vi "Set Visible State.vi"(6 "Event Structure Frame (-1: Use State Name)":i32=-1, 7 "Event Structure (F: Case Structure)":bool, 8 "error in (no error)":errorcluster, 9 "State Name":string, 10 "Category (Optional)":string, 11 "JKI SM in":refnum<class "JKI SM.lvclass">) -> (0 "error out":errorcluster, 3 "JKI SM out":refnum<class "JKI SM.lvclass">)   [LabVIEW 2020, in "JKI State Machine API.lvlib" / "JKI SM.lvclass"]
uses:
  JKI SM.lvclass
  JKI SM.lvclass/JKI SM.ctl
  <userlib>/_OpenG.lib/string/string.llb/Trim Whitespace (String Array)__ogtk.vi
  <userlib>/_OpenG.lib/string/string.llb/Trim Whitespace (String)__ogtk.vi
  <userlib>/_OpenG.lib/string/string.llb/openg_string.lvlib
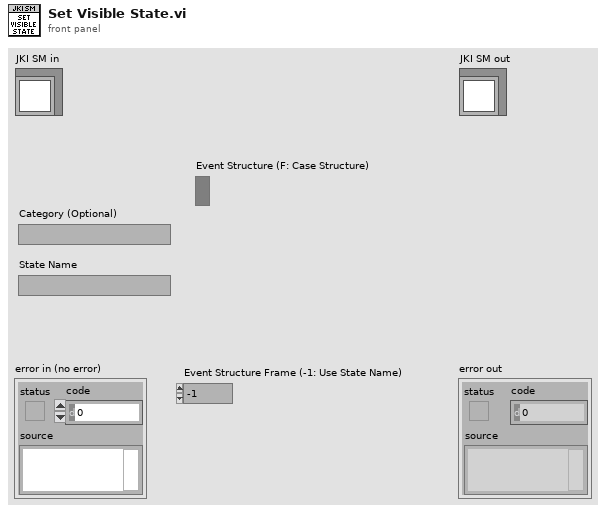
[diagram p1: front panel]
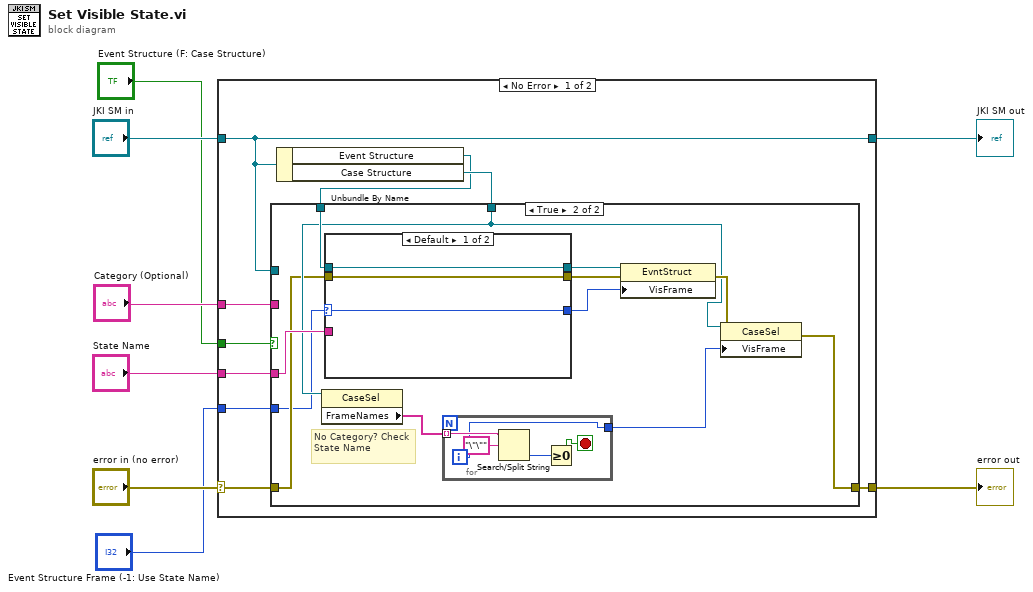
[diagram p0: block diagram]
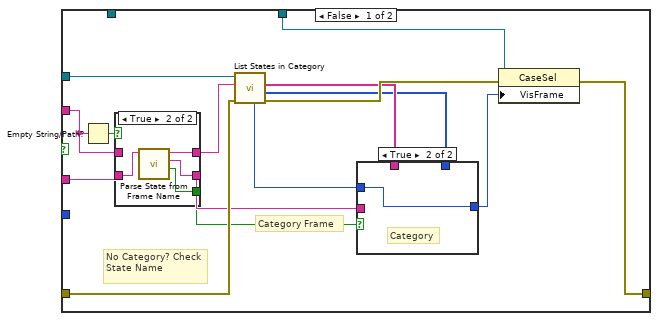
[diagram p2: hidden frame]
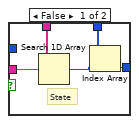
[diagram p3: hidden frame]
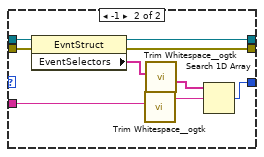
[diagram p5: hidden frame]
diagram:
  n1 = case shown="No Error" "error in (no error)" {
    selector: "error in (no error)" -> [w12 w75]
    tunnel: [w17 w75] -> w7
    tunnel: [w13 w74] -> w5
    tunnel: "JKI SM in" -> [w13 w74]
    tunnel: "State Name" -> [w14 _]
    tunnel: "Category (Optional)" -> [w15 _]
    tunnel: "Event Structure (F: Case Structure)" -> [w11 _]
    tunnel: "Event Structure Frame (-1: Use State Name)" -> [w9 _]
    frame No Error {
      n2 = Unbundle By Name(w13) -> ("Event Structure"=w10:refnum<vi>, "Case Structure"=w16:refnum<vi>)
      n3 = case shown="True" w11 {
        tunnel: [w32 w51] -> w17
        tunnel: w16 -> [w31 w50]
        tunnel: w15 -> [w28 _]
        tunnel: w14 -> [w27 w56]
        tunnel: w13 -> [w26 _]
        tunnel: w12 -> [w25 w47]
        tunnel: w10 -> [_ w54]
        tunnel: w9 -> [_ w45]
        frame False {
          # "Category Frame"
          # "No Category? Check State Name"
          n4 = Empty String/Path?(string/path=w28) -> (empty?=w29:bool)
          n5 = case shown="True" w29 {
            tunnel: w27 -> [w39 w44]
            tunnel: [w40 w43] -> w24
            tunnel: w28 -> [w40 _]
            tunnel: [w39 w42] -> w22
            tunnel: [_ w41] -> w19
            frame False {
            }
            frame True {
              n6 = call "Parse State from Frame Name.vi"("Frame or State Name"=w44) -> ("is a Category Frame?"=w41:bool, "State Name"=w42:string, "Category Name"=w43:string)  [unwired: 5 in, 3 out]
            }
          }
          n7 = call "List States in Category.vi"("error in (no error)"=w25, "Category"=w24, "JKI SM in"=w26) -> ("error out"=w30:errorcluster, "State Frame Indices"=w21:i32[], "States"=w23:string[], "Category Frame Index"=w18:i32)  [unwired: 4 in, 1 out]
          n8 = case shown="True" w19 {
            tunnel: w23 -> [w37 _]
            tunnel: w22 -> [w36 _]
            tunnel: w21 -> [w35 _]
            tunnel: [w33 w38] -> w20
            tunnel: w18 -> [_ w38]
            frame False {
              # "State"
              n9 = Search 1D Array(1D array=w37, element=w36) -> (index of element=w34:i32)  [unwired: 1 in]
              n10 = Index Array(array=w35, index=w34) -> (element=w33:i32)
            }
            frame True {
              # "Category"
            }
          }
          n11 = property class="CaseSel"(reference=w31, error in=w30, "VisFrame"=w20) -> (error out=w32:errorcluster)  [unwired: 1 out]
        }
        frame True {
          # "No Category? Check State Name"
          n12 = property class="CaseSel"(reference=w50) -> ("FrameNames"=w49:string[])  [unwired: 1 in, 2 out]
          n13 = case shown="Default" w45 {
            selector: w45 -> [w58 _]
            tunnel: w56 -> [_ w68]
            tunnel: [w58 w67] -> w55
            tunnel: w54 -> [w59 w66]
            tunnel: [w59 w64] -> w53
            tunnel: w47 -> [w57 w61]
            tunnel: [w57 w60] -> w46
            frame Default {
            }
            frame -1 {
              n14 = property class="EvntStruct"(reference=w66, error in=w61) -> (reference out=w64:refnum<vi>, error out=w60:errorcluster, "EventSelectors"=w65:string[])
              n15 = call-poly <userlib>:"Trim Whitespace__ogtk.vi"("String in"=w68) -> ("String out"=w62:string)  [unwired: 6 in]
              n16 = call-poly <userlib>:"Trim Whitespace__ogtk.vi"("String in"=w65) -> ("String out"=w63:string[])  [unwired: 6 in]
              n17 = Search 1D Array(1D array=w63, element=w62) -> (index of element=w67:i32)  [unwired: 1 in]
            }
          }
          n18 = for {
            tunnel: w49 -> [w73] mode=indexing
            tunnel: [w70] -> w48
            i -> [w70]
            stop <- w69 stop-if-true
            n19 = Search/Split String(string=w73, search string/char (-)="\"\"") -> (offset of match=w71:i32)  [unwired: 1 in, 2 out]
            n20 = Greater Or Equal To 0?(x=w71) -> (x >= 0?=w69:bool)
          }
          n21 = property class="EvntStruct"(reference=w53, error in=w46, "VisFrame"=w55) -> (error out=w52:errorcluster)  [unwired: 1 out]
          n22 = property class="CaseSel"(reference=w50, error in=w52, "VisFrame"=w48) -> (error out=w51:errorcluster)  [unwired: 1 out]
        }
      }
    }
    frame Error {
    }
  }
  "error out" <- w7
  "JKI SM out" <- w5
